vi "Create Data Channel_ex.vi"() -> ()   [LabVIEW 2019]
uses:
  <vilib>/NI VeriStand/Custom Device API/Custom Device Item Ref.ctl
  Control 14.ctl
  Scripting API/Polymorphic/Create Channel/Create Response Single Channel_Comparison.vi
  Scripting API/Scripting API.lvlib
  <vilib>/NI VeriStand/Custom Device API/Custom Device API.lvlib
panel:
  out "Message Refnum Out":T1=18446744073709551615 format="%.0x"
  out "Channel Refnum":T1=18446744073709551615 format="%.0x"
  out "Error Out":errorcluster
  in  "Message Refnum In":T1=18446744073709551615 format="%.0x"
  in  "Error In":errorcluster
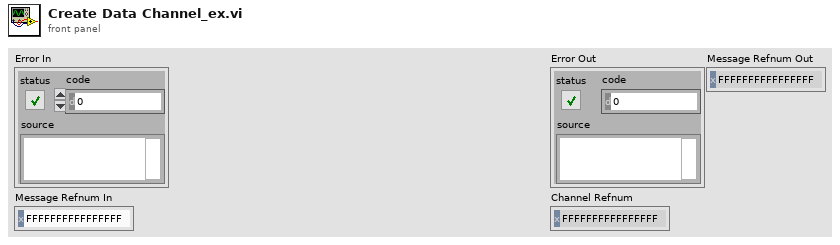
[diagram p1: front panel]
types:
  T1 = typedef "Custom Device API.lvlib/Custom Device Item Ref.ctl" = u64
  T2 = typedef "Control 14.ctl" = cluster{"Expected String":string, "Default Value":dbl, "Units":string}
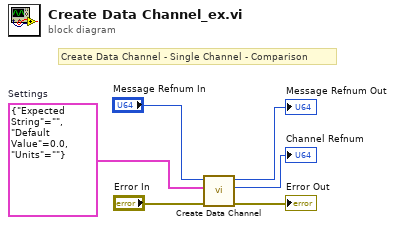
[diagram p0: block diagram]
diagram:
  w1 = T2 {"Expected String"="", "Default Value"=0.0, "Units"=""}  # Settings
  # "Create Data Channel - Single Channel - Comparison"
  n1 = call-poly "Create Data Channel.vi"("Error In"="Error In", "Settings"=w1, "Message Refnum In"="Message Refnum In") -> ("Error Out"=→"Error Out":errorcluster, "Channel Refnum"=→"Channel Refnum":T1, "Message Refnum Out"=→"Message Refnum Out":T1)  [unwired: 6 in]
